vi "Shared stop.vi"(11 "stop":bool) -> (3 "stop 2":bool)   [LabVIEW 2021]
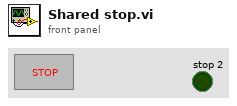
[diagram p1: front panel]
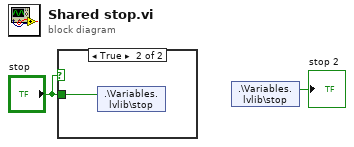
[diagram p0: block diagram]
diagram:
  n1 = case shown="True" "stop" {
    tunnel: "stop" -> [_ w3]
    frame False {
    }
    frame True {
      n2 = shared-variable ".\\Variables.lvlib\\stop"(w3) -> ()  [unwired: 1 in, 1 out]
    }
  }
  n3 = shared-variable ".\\Variables.lvlib\\stop"() -> (→"stop 2":bool)  [unwired: 1 in, 1 out]
